vi "populateModelSettings.vi"(8 "error in (no error)":errorcluster, 10 "Model in":refnum<class "Model.lvclass">, 11 "Boot in":refnum<class "Boot.lvclass">) -> (0 "error out":errorcluster, 2 "Model out":refnum<class "Model.lvclass">, 3 "Boot out":refnum<class "Boot.lvclass">)   [LabVIEW 2016, in "Boot.lvclass"]
uses:
  Boot.lvclass
  Model/Model.lvclass
  Model/Model.lvclass/Model.ctl
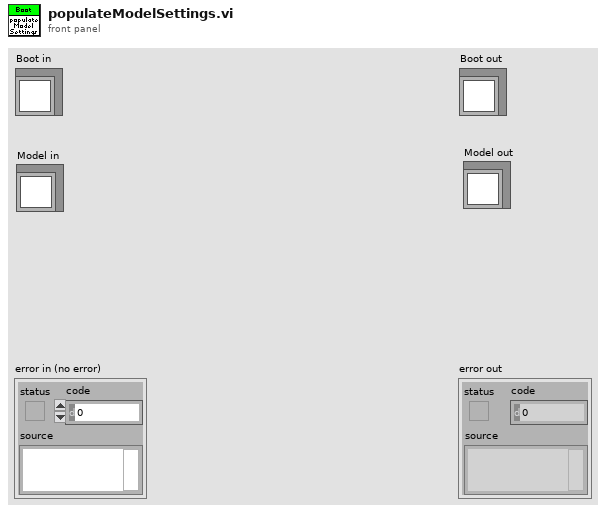
[diagram p1: front panel]
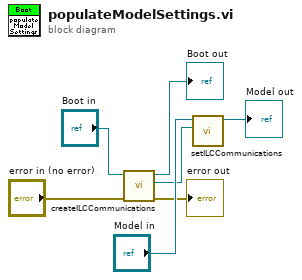
[diagram p0: block diagram]
diagram:
  n1 = call "createILCCommunications.vi"("error in (no error)"="error in (no error)", "Boot in"="Boot in") -> ("error out"=→"error out":errorcluster, "ILCCommunications"=w5:refnum<class "ILCCommunications.lvclass">, "Boot out"=→"Boot out":refnum<class "Boot.lvclass">)  [unwired: 7 in]
  n2 = call "setILCCommunications.vi"("ILCCommunications"=w5, "Model in"="Model in") -> ("Model out"=→"Model out":refnum<class "Model.lvclass">)  [unwired: 9 in]
